vi "XML - Get absolute RT Driver VI path for TARGET.vi"(7 "Target Type (Windows)":T1, 8 "error in (no error)":errorcluster, 11 "CD Wizard - Internal Data":T2) -> (0 "error out":errorcluster, 3 "Relative RT Driver TARGET path":path)   [LabVIEW 2015]
doc: "Create the absolute path for the RT Driver VI inside the Configuration LLB for the <B>RT Target</B> based on the name and execution mode of the new custom device."
uses:
  TypDef/CD Wizard - Internal data.ctl
  TypDef/CD Wizard - Execution Mode.ctl
  TypDef/CD Wizard - Extra Page Name and GUID.ctl
  TypDef/Target Type.ctl
  Constants/Constants TypDef/CD Engine lvlib.ctl
  Constants/Constants TypDef/Build Spec Engine.ctl
  Constants/Build Spec Engine.vi
  Constants/CD Engine lvlib.vi
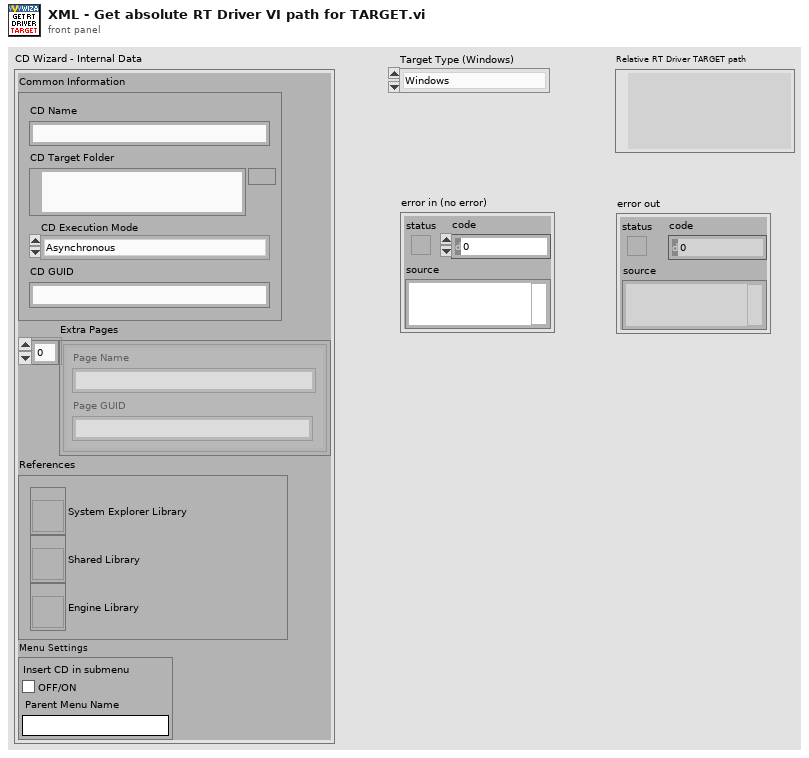
[diagram p1: front panel]
types:
  T1 = typedef "Target Type.ctl" = enum16{"Windows", "VxWorks", "Pharlap", "Linux 32 ARM", "Linux x64"}
  T2 = typedef "CD Wizard - Internal data.ctl" = cluster{"Common Information":cluster{"CD Name":string, "CD Target Folder":path, "CD Execution Mode":T3, "CD GUID":string}, "Extra Pages":T4[], "References":cluster{"System Explorer Library":refnum<vi>, "Shared Library":refnum<vi>, "Engine Library":refnum<vi>}, "Menu Settings":cluster{"Insert CD in submenu":bool, "Parent Menu Name":string}}
  T3 = typedef "CD Wizard - Execution Mode.ctl" = enum16{"Asynchronous", "Inline HW Interface", "Inline Model Interface", "Inline Timing and Sync", "Asynchronous Timing and Sync"}
  T4 = typedef "CD Wizard - Extra Page Name and GUID.ctl" = cluster{"Page Name":string, "Page GUID":string}
  T5 = typedef "CD Engine lvlib.ctl" = enum16{"LibraryFileName", "LibraryFolderName", "Engine.FolderName", "Engine.Init.FolderName", "Engine.Run.FolderName", "Engine.Shutdown.FolderName", "Types.FolderName", "Engine.RT Driver VI.TemplatePath", "Engine.RT Driver VI.FileName"}
  T6 = typedef "Build Spec Engine.ctl" = enum16{"Destinations.LLBWindowsFileName", "Destinations.LLBVxWorksFileName", "Destinations.LLBPharlapFileName", "Destinations.LLBLinuxARMFileName", "Destinations.LLBLinux64FileName"}
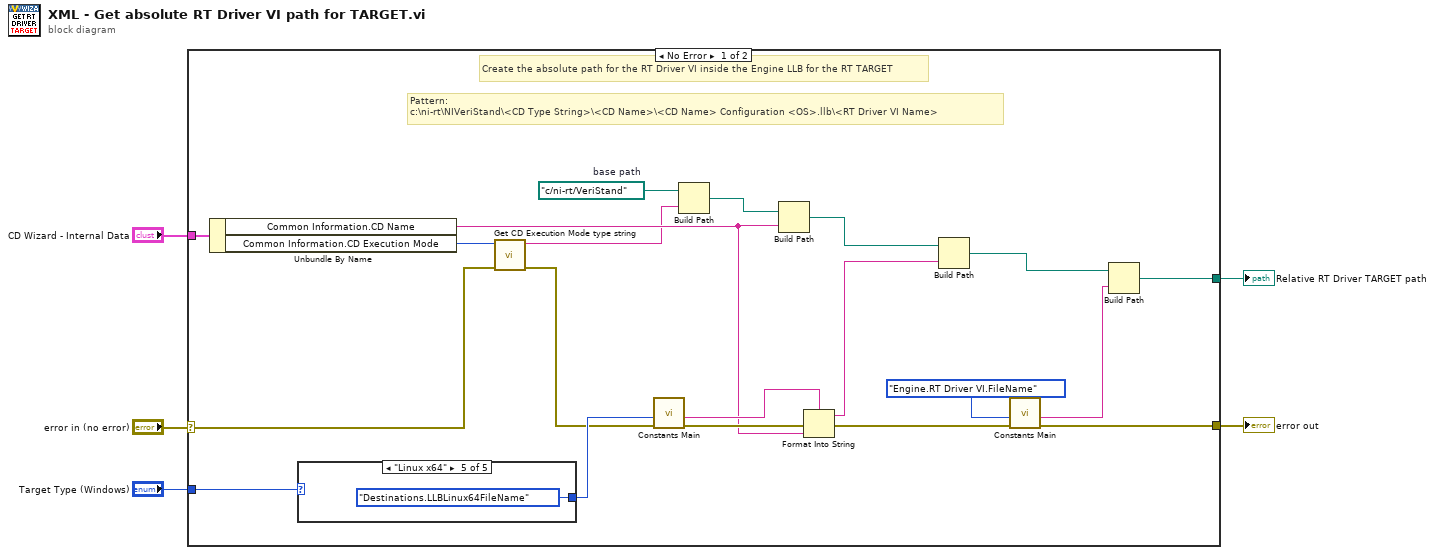
[diagram p0: block diagram]
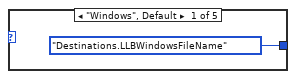
[diagram p2: hidden frame]
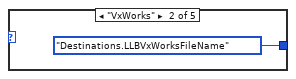
[diagram p3: hidden frame]
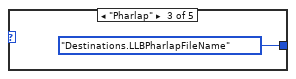
[diagram p4: hidden frame]
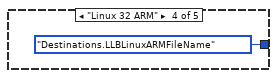
[diagram p5: hidden frame]
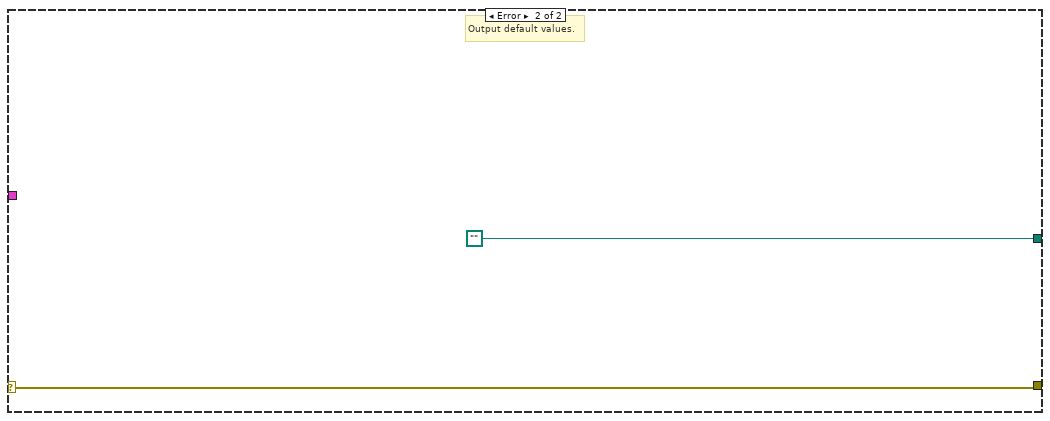
[diagram p6: hidden frame]
diagram:
  n1 = case shown="No Error" "error in (no error)" {
    selector: "error in (no error)" -> [w17 w32]
    tunnel: [w7 w32] -> w2
    tunnel: [w9 path ""] -> w4
    tunnel: "CD Wizard - Internal Data" -> [w22 _]
    tunnel: "Target Type (Windows)" -> [w20 _]
    frame No Error {
      w15 = path "c:/ni-rt/VeriStand"  # base path
      # "Pattern:\nc:\\ni-rt\\NIVeriStand\\<CD Type String>\\<CD Name>\\<CD Name> Configuration <OS>.llb\\<RT Driver VI Name>"
      # "Create the absolute path for the RT Driver VI inside the Engine LLB for the RT TARGET"
      n2 = Unbundle By Name(w22) -> ("Common Information.CD Name"=w14:string, "Common Information.CD Execution Mode"=w18:T3)
      n3 = case shown="\"Linux x64\"" w20 {
        tunnel: [Build_Spec_Engine."Destinations.LLBWindowsFileName" ("Action") Build_Spec_Engine."Destinations.LLBVxWorksFileName" ("Action") Build_Spec_Engine."Destinations.LLBPharlapFileName" ("Action") Build_Spec_Engine."Destinations.LLBLinuxARMFileName" ("Action") Build_Spec_Engine."Destinations.LLBLinux64FileName" ("Action")] -> w19
        frame "Windows", Default {
        }
        frame "VxWorks" {
        }
        frame "Pharlap" {
        }
        frame "Linux 32 ARM" {
        }
        frame "Linux x64" {
        }
      }
      n4 = call "Get CD Execution Mode type string.vi"("error in (no error)"=w17, "CD Execution Mode"=w18) -> ("error out"=w16:errorcluster, "Execution Mode type"=w13:string)  [unwired: 8 in]
      n5 = call-poly "Constants Main.vi"("error in (no error)"=w16, "Action"=w19) -> ("error out"=w23:errorcluster, "Output"=w24:string)  [unwired: 8 in]
      n6 = Build Path(base path=w15, name or relative path=w13) -> (appended path=w12:path)
      n7 = Build Path(base path=w12, name or relative path=w14) -> (appended path=w21:path)
      n8 = Format Into String(format string=w24, error in=w23, w14) -> (resulting string=w25:string, error out=w8:errorcluster)  [unwired: 1 in]
      n9 = Build Path(base path=w21, name or relative path=w25) -> (appended path=w10:path)
      n10 = call-poly "Constants Main.vi"("error in (no error)"=w8, "Action"=CD_Engine_lvlib."Engine.RT Driver VI.FileName") -> ("error out"=w7:errorcluster, "Output"=w6:string)  [unwired: 8 in]
      n11 = Build Path(base path=w10, name or relative path=w6) -> (appended path=w9:path)
    }
    frame Error {
      # "Output default values."
    }
  }
  "error out" <- w2
  "Relative RT Driver TARGET path" <- w4
